vi "Day 6.1 - generations.vi"(11 "input":string[](array[string])) -> (3 "output":u32)   [LabVIEW 2021]
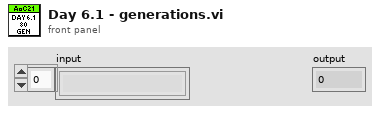
[diagram p1: front panel]
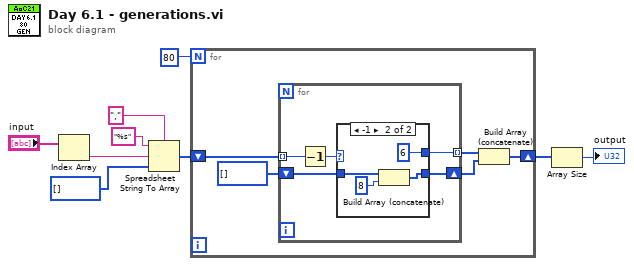
[diagram p0: block diagram]
diagram:
  n1 = Index Array(array="input") -> (element=w8:string)  [unwired: 1 in]
  n2 = Spreadsheet String To Array(delimiter (Tab)=",", format string="%s", spreadsheet string=w8, array type (2D Dbl)=i32[] []) -> (array=w4:i32[])
  n3 = for {
    N: 80 -> [_]
    shift-right: [w10] -> w2
    shift-left: w4 -> [w14]
    n4 = for {
      tunnel: w14 -> [w19] mode=indexing
      tunnel: [w16] -> w12 mode=indexing
      shift-right: [w17] -> w11
      shift-left: i32[] [] -> [w18]
      n5 = Decrement(x=w19) -> (x-1=w15:i32)
      n6 = case shown="-1" w15 {
        selector: w15 -> [w20 _]
        tunnel: w18 -> [w21 w25]
        tunnel: [w21 w24] -> w17
        tunnel: [w20 6] -> w16
        frame 0, Default {
        }
        frame -1 {
          n7 = Build Array (concatenate)(w25, 8) -> (w24:i32[])
        }
      }
    }
    n8 = Build Array (concatenate)(w12, w11) -> (w10:i32[])
  }
  n9 = Array Size(array=w2) -> (size(s)=→"output":i32)
